vi "Set Parameters (uSMC).vi"(8 "error in (no error)":errorcluster, 9 "Index":i32, 11 "Visa array in":refnum<visa-resource-name>[](array[refnum])) -> (0 "error out":errorcluster, 3 "Visa Array out":refnum<visa-resource-name>[](array[refnum]))   [LabVIEW 2010, in "SignalWriterMH110203USBStepperMotor.lvclass"]
uses:
  SignalWriterMH110203USBStepperMotor.lvclass
  class_data.vi
panel:
  out "array buffer":u8[](array[numeric])
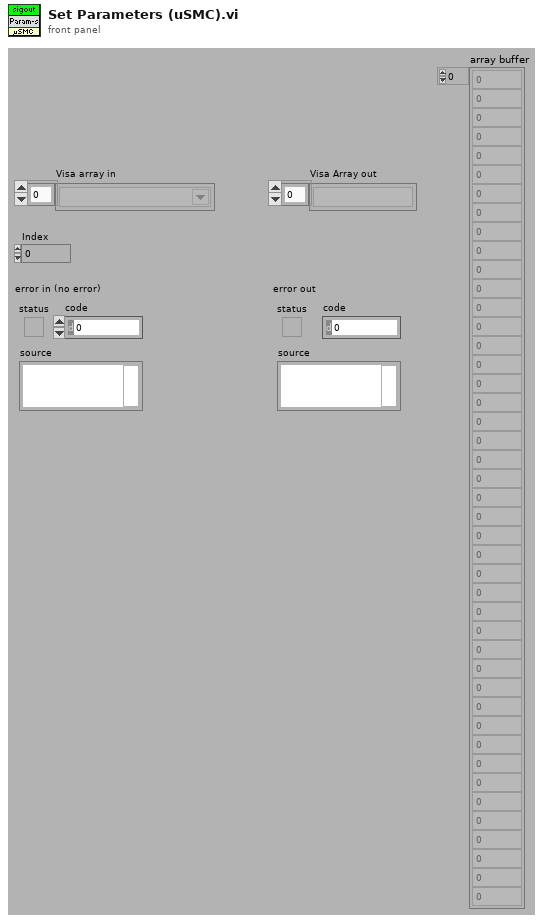
[diagram p1: front panel]
types:
  T1 = typedef "SignalWriterMH110203USBStepperMotor.lvclass/Set Parameters (uSMC).ctl" = cluster{"Acceleration Time":u8, "Deceleration Time":u8, "Reduce Current Timeout":u16, "Buttons Timeout 1":u16, "Buttons Timeout 2":u16, "Buttons Timeout 3":u16, "Buttons Timeout 4":u16, "Buttons Timeout Reset":u16, "Buttons Timeout DblClick":u16, "Reset Speed":u16, "Buttons Speed 1":u16, "Buttons Speed 2":u16, "Buttons Speed 3":u16, "Buttons Speed 4":u16, "Max Backlash":u16, "Start Pos":i32, "RTdelta":u16, "RTMinError":u16, "Maximum Temperature":u16, "Sync Duration":u8, "Backlash Speed":u16, "EncVSCP":u8, "Steps Per Revolution":i32, "Encoder Pulses Per Rev-on":i32}
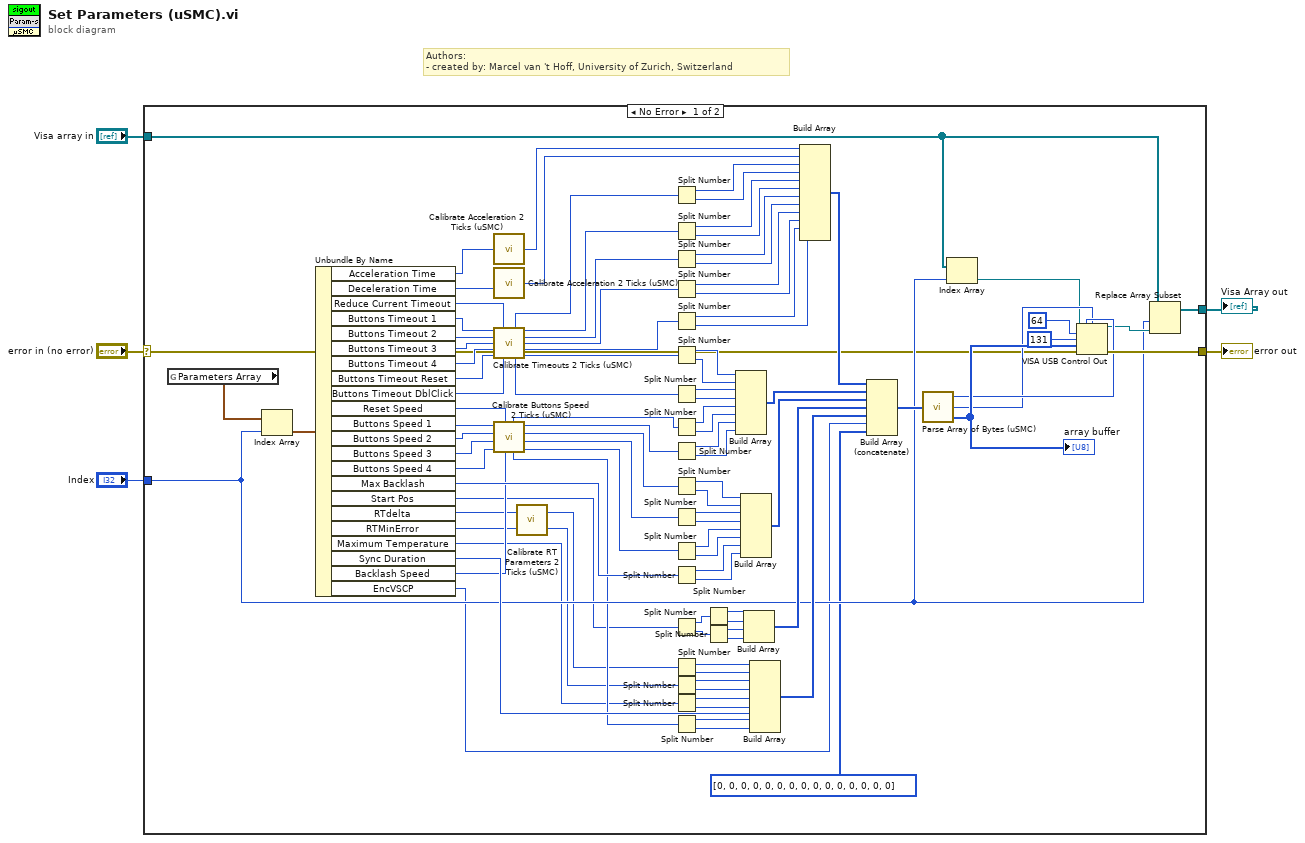
[diagram p0: block diagram]
diagram:
  # "Authors: \n- created by: Marcel van 't Hoff, University of Zurich, Switzerland"
  n1 = case shown="No Error" "error in (no error)" {
    selector: "error in (no error)" -> [w7 w107]
    tunnel: [w103 w107] -> w5
    tunnel: [w52 w106] -> w4
    tunnel: "Index" -> [w46 _]
    tunnel: "Visa array in" -> [w6 w106]
    frame No Error {
      n2 = global read "class_data.vi" "Parameters Array"() -> (w50:T1[])
      n3 = Index Array(array=w50, index=w46) -> (element=w49:T1)
      n4 = Unbundle By Name(w49) -> ("Acceleration Time"=w45:u8, "Deceleration Time"=w43:u8, "Reduce Current Timeout"=w41:u16, "Buttons Timeout 1"=w40:u16, "Buttons Timeout 2"=w39:u16, "Buttons Timeout 3"=w38:u16, "Buttons Timeout 4"=w37:u16, "Buttons Timeout Reset"=w36:u16, "Buttons Timeout DblClick"=w35:u16, "Reset Speed"=w27:u16, "Buttons Speed 1"=w26:u16, "Buttons Speed 2"=w25:u16, "Buttons Speed 3"=w19:u16, "Buttons Speed 4"=w18:u16, "Max Backlash"=w55:u16, "Start Pos"=w8:i32, "RTdelta"=w11:u16, "RTMinError"=w12:u16, "Maximum Temperature"=w13:u16, "Sync Duration"=w54:u8, "Backlash Speed"=w17:u16, "EncVSCP"=w14:u8)
      n5 = call "Calibrate Acceleration 2 Ticks (uSMC).vi"("Acceleration Value"=w45) -> ("Acceleration ticks"=w44:u8)
      n6 = call "Calibrate Acceleration 2 Ticks (uSMC).vi"("Acceleration Value"=w43) -> ("Acceleration ticks"=w42:u8)
      n7 = call "Calibrate Timeouts 2 Ticks (uSMC).vi"("Buttons Timeout 1 (ms)"=w40, "Reduce Current Timeout (ms)"=w41, "Buttons Timeout 2 (ms)"=w39, "Buttons Timeout 3 (ms)"=w38, "Buttons Timeout 4 (ms)"=w37, "Buttons Timeout Reset (ms)"=w36, "Buttons Timeout DblClick (ms)"=w35) -> ("Reduce Current Timeout (ticks)"=w28:u16, "Buttons Timeout 1 (ticks)"=w29:u16, "Buttons Timeout 2 (ticks)"=w30:u16, "Buttons Timeout 3 (ticks)"=w31:u16, "Buttons Timeout 4 (ticks)"=w32:u16, "Buttons Timeout DblClick (ticks)"=w34:u16, "Buttons Timeout Reset (ticks)"=w33:u16)  [unwired: 2 in]
      n8 = call "Calibrate Buttons Speed 2 Ticks (uSMC).vi"("Backlash Speed (Full Steps/Sec)"=w17, "Reset Speed (Full Steps/Sec)"=w27, "Buttons Speed 4 (Full Steps/Sec)"=w18, "Buttons Speed 3 (Full Steps/Sec)"=w19, "Buttons Speed 2 (Full Steps/Sec)"=w25, "Buttons Speed 1 (Full Steps/Sec)"=w26) -> ("Buttons Speed 4 (ticks)"=w20:u16, "Buttons Speed 3 (ticks)"=w21:u16, "Buttons Speed 2 (ticks)"=w22:u16, "Buttons Speed 1 (ticks)"=w23:u16, "Backlash Speed (ticks)"=w16:u16, "Reset Speed (ticks)"=w24:u16)
      n9 = call "Calibrate RT Parameters 2 Ticks (uSMC).vi"("RTMinError (a.u.)"=w12, "RTDelta (a.u.)"=w11) -> ("RTMinError (ticks)"=w9:u16, "RTDelta (ticks)"=w10:u16)
      n10 = Split Number(x=w28) -> (hi(x)=w102:u8, lo(x)=w101:u8)
      n11 = Split Number(x=w29) -> (hi(x)=w100:u8, lo(x)=w99:u8)
      n12 = Split Number(x=w30) -> (hi(x)=w98:u8, lo(x)=w97:u8)
      n13 = Split Number(x=w31) -> (hi(x)=w96:u8, lo(x)=w95:u8)
      n14 = Split Number(x=w32) -> (hi(x)=w94:u8, lo(x)=w93:u8)
      n15 = Split Number(x=w33) -> (hi(x)=w92:u8, lo(x)=w91:u8)
      n16 = Split Number(x=w34) -> (hi(x)=w90:u8, lo(x)=w89:u8)
      n17 = Split Number(x=w24) -> (hi(x)=w88:u8, lo(x)=w87:u8)
      n18 = Split Number(x=w23) -> (hi(x)=w86:u8, lo(x)=w85:u8)
      n19 = Split Number(x=w22) -> (hi(x)=w77:u8, lo(x)=w78:u8)
      n20 = Split Number(x=w21) -> (hi(x)=w79:u8, lo(x)=w80:u8)
      n21 = Split Number(x=w20) -> (hi(x)=w81:u8, lo(x)=w82:u8)
      n22 = Split Number(x=w55) -> (hi(x)=w83:u8, lo(x)=w84:u8)
      n23 = Split Number(x=w8) -> (hi(x)=w76:u16, lo(x)=w75:u16)
      n24 = Split Number(x=w10) -> (hi(x)=w62:u8, lo(x)=w61:u8)
      n25 = Split Number(x=w9) -> (hi(x)=w60:u8, lo(x)=w59:u8)
      n26 = Split Number(x=w13) -> (hi(x)=w58:u8, lo(x)=w57:u8)
      n27 = Split Number(x=w16) -> (hi(x)=w48:u8, lo(x)=w47:u8)
      n28 = Split Number(x=w76) -> (hi(x)=w74:u8, lo(x)=w73:u8)
      n29 = Split Number(x=w75) -> (hi(x)=w72:u8, lo(x)=w71:u8)
      n30 = Build Array(w92, w91, w90, w89, w88, w87, w86, w85) -> (w69:u8[])
      n31 = Build Array(w77, w78, w79, w80, w81, w82, w83, w84) -> (w68:u8[])
      n32 = Build Array(w74, w73, w72, w71) -> (w67:u8[])
      n33 = Build Array(w62, w61, w60, w59, w58, w57, w54, w48, w47) -> (w56:u8[])
      n34 = Build Array(w44, w42, w102, w101, w100, w99, w98, w97, w96, w95, w94, w93) -> (w70:u8[])
      n35 = Build Array (concatenate)(w70, w69, w68, w67, w56, w14, u8[] [0, 0, 0, 0, 0, 0, 0, 0, 0, 0, 0, 0, 0, 0, 0] ("initialized array")) -> (w66:u8[])
      n36 = call "Parse Array of Bytes (uSMC).vi"("byte array"=w66) -> ("first 2 bytes"=w64:u16, "second 2 bytes"=w63:u16, "array buffer"=w65:u8[])
      "array buffer" <- w65
      n37 = Index Array(array=w6, index=w46) -> (element=w53:refnum<visa-resource-name>)
      n38 = VISA USB Control Out(0:w53, 1:w64, 2:w63, 5:i16 64 ("request type"), 7:i16 131 ("request type"), 9:w65, 11:w7) -> (4:w51:refnum<visa-resource-name>, 15:w103:errorcluster)
      n39 = Replace Array Subset(array=w6, new element=w51, index=w46) -> (w52:refnum<visa-resource-name>[])
    }
    frame Error {
    }
  }
  "error out" <- w5
  "Visa Array out" <- w4
